vi "B_GetProperty.vi"(0 "reference in":refnum<class "Child.lvclass">, 5 "error in (no error)":errorcluster) -> (14 "reference out":refnum<class "Child.lvclass">, 15 "property":dbl, 19 "error out":errorcluster)   [LabVIEW 2019, in "Child.lvclass"]
uses:
  Child.lvclass
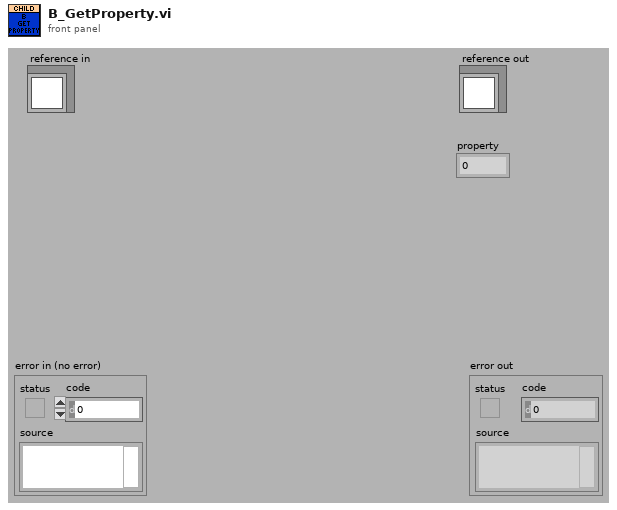
[diagram p1: front panel]
types:
  T1 = typedef "Child.lvclass/ObjectAttributes.ctl" = cluster{"Attribute0":dbl}
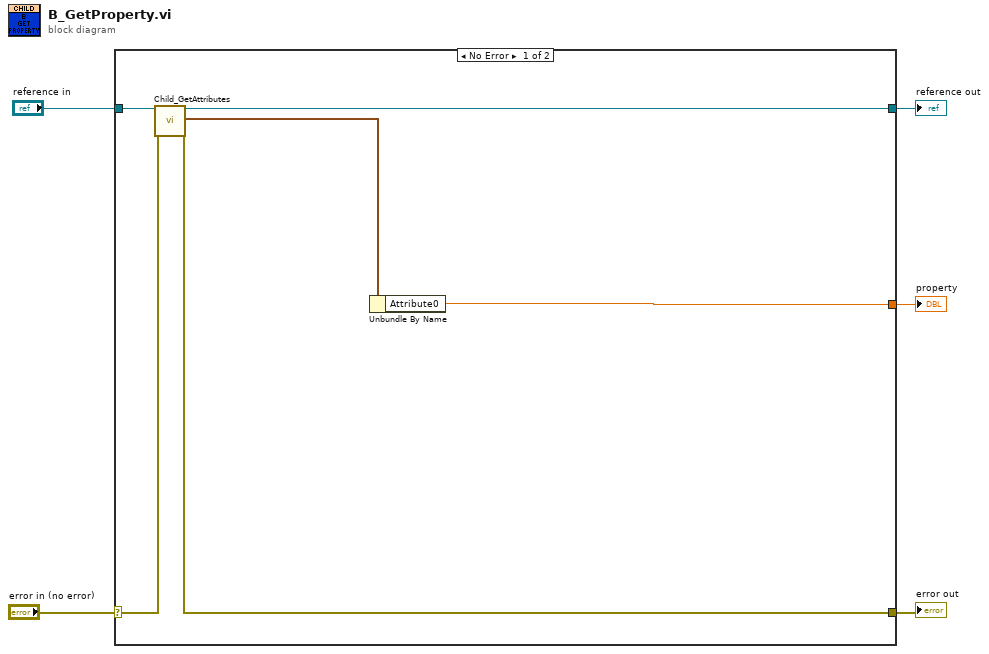
[diagram p0: block diagram]
diagram:
  n1 = case shown="No Error" "error in (no error)" {
    selector: "error in (no error)" -> [w11 w13]
    tunnel: [w10 w13] -> w4
    tunnel: [w8 w12] -> w2
    tunnel: "reference in" -> [w9 w12]
    tunnel: [w7 _] -> w1
    frame No Error {
      n2 = call "Child_GetAttributes.vi"("reference in"=w9, "error in (no error)"=w11) -> ("reference out"=w8:refnum<class "Child.lvclass">, "Data"=w6:T1, "error out"=w10:errorcluster)  [unwired: 14 in, 1 out]
      n3 = Unbundle By Name(w6) -> ("Attribute0"=w7:dbl)
    }
    frame Error {
    }
  }
  "error out" <- w4
  "reference out" <- w2
  "property" <- w1
